vi "SendSetDigitalPWMCommand.vi"(2 "Value [0 - 255]":u8=1, 3 "Pin [0 - 11]":u8=1 max=11, 4 "Port Distant":u16, 5 "Addresse IP":u32, 6 "entrée d'erreur (pas d'erreur)":errorcluster, 7 "Connexion réseau UDP en entrée":refnum<k16>) -> (0 "sortie d'erreur":errorcluster, 1 "Connexion réseau UDP en sortie":refnum<k16>)   [LabVIEW 2021]
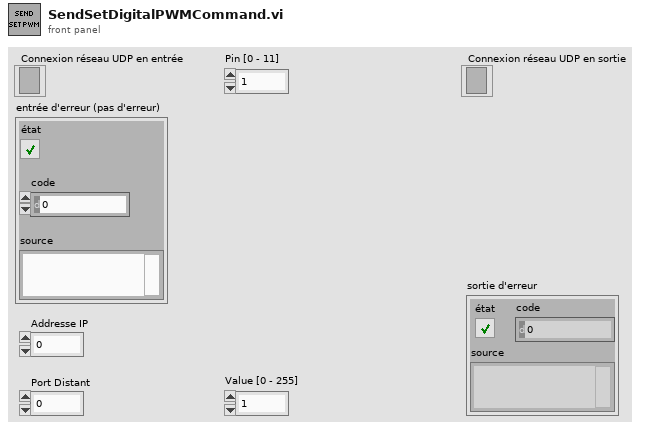
[diagram p1: front panel]
types:
  T1 = typedef "CommandType.ctl" = u8[]
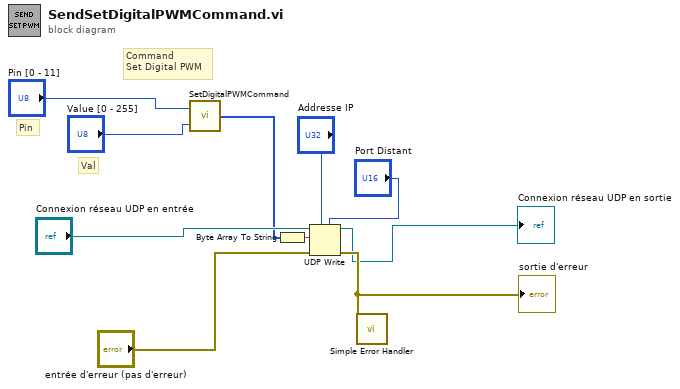
[diagram p0: block diagram]
diagram:
  # "Command \nSet Digital PWM"
  # "Val"
  # "Pin"
  n1 = call "SetDigitalPWMCommand.vi"("Value"="Value [0 - 255]", "Pin"="Pin [0 - 11]") -> ("Command"=w1:T1)
  n2 = Byte Array To String(unsigned byte array=w1) -> (string=w5:string)
  n3 = UDP Write(address="Addresse IP", port or service name="Port Distant", connection ID="Connexion réseau UDP en entrée", data in=w5, 8:"entrée d'erreur (pas d'erreur)") -> (error out=w6:errorcluster, 3:→"Connexion réseau UDP en sortie":refnum<k16>)  [unwired: 1 in]
  "sortie d'erreur" <- w6
  n4 = call <vilib>:"Simple Error Handler.vi"("error in (no error)"=w6) -> ()  [unwired: 4 in, 5 out]
